vi "RateLimitWhenSpeedingUp.vi"(10 "Ramp":dbl=1.0, 11 "Input":dbl(slide) scale=-1.0..1.0) -> (3 "Output":dbl(slide) scale=-1.0..1.0)   [LabVIEW 2016]
doc: "Limits how fast the input changes, only when the magnitude of the input is increasing"
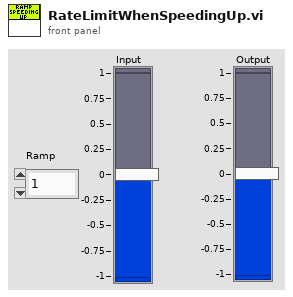
[diagram p1: front panel]
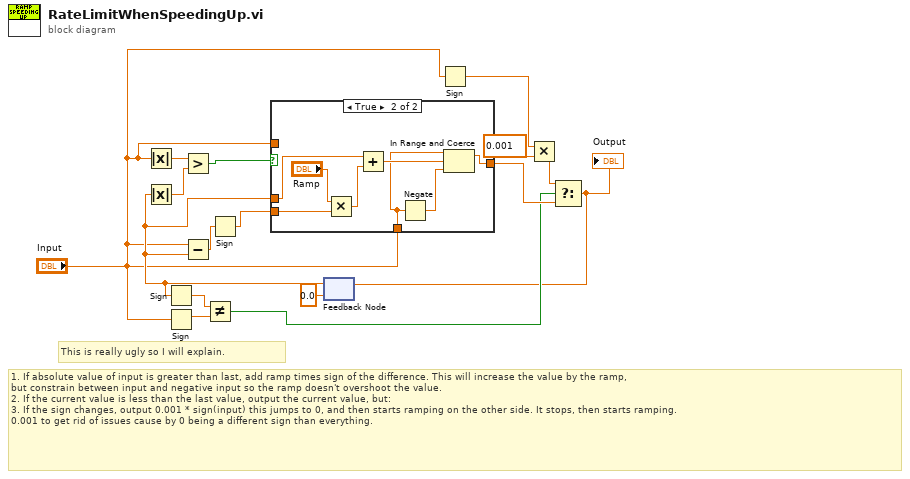
[diagram p0: block diagram]
diagram:
  # "1. If absolute value of input is greater than last, add ramp times sign of the difference. This will increase the value by the ramp,\nbut constrain between input and negative input so the ramp doesn't overshoot the value. \n2. If the current value is less than the last value, output the current value, but:\n3. If the sign changes, output 0.001 * sign(input) this jumps to 0, and then starts ramping on the other side. It stops, then starts ramping.\n0.001 to get rid of issues cause by 0 being a different sign than everything."
  # "This is really ugly so I will explain."
  n1 = Absolute Value(x="Input") -> (abs(x)=w16:dbl)
  n2 = Sign(1:"Input") -> (0:w10:dbl)
  n3 = feedback #1(0.0 ("Input")) -> (w8:dbl)
  n4 = Absolute Value(x=w8) -> (abs(x)=w15:dbl)
  n5 = Sign(1:w8) -> (0:w11:dbl)
  n6 = Greater?(x=w16, y=w15) -> (0:w14:bool)
  n7 = Subtract(x="Input", y=w8) -> (x-y=w12:dbl)
  n8 = Not Equal?(x=w11, y=w10) -> (x != y?=w7:bool)
  n9 = Sign(1:w12) -> (0:w13:dbl)
  n10 = case shown="True" w14 {
    tunnel: [w17 w20] -> w9
    tunnel: w13 -> [_ w24]
    tunnel: w8 -> [_ w22]
    tunnel: "Input" -> [w17 _]
    tunnel: "Input" -> [_ w19]
    frame False {
    }
    frame True {
      n11 = Multiply(x="Ramp", y=w24) -> (x*y=w25:dbl)
      n12 = Add(x=w22, y=w25) -> (x+y=w21:dbl)
      n13 = Negate(x=w19) -> (-x=w18:dbl)
      n14 = In Range and Coerce(upper limit=w19, x=w21, lower limit=w18) -> (coerced(x)=w20:dbl)  [unwired: 1 out]
    }
  }
  n15 = Sign(1:"Input") -> (0:w4:dbl)
  n16 = Multiply(x=w4, y=0.001) -> (x*y=w6:dbl)
  n17 = Select(t=w6, s=w7, f=w9) -> (s? t:f=w3:dbl)
  "Output" <- w3
  n18 = feedback-in #1(w3) -> ()
